vi "Asylum_Driver_LithographyObjects.vi"(4 "Abort Notifier":refnum<notifier>, 5 "Writing Setpoint":dbl=0.1 format="%#_13g", 6 "Interpolation":dbl format="%#_13g", 7 "Move Setpoint":dbl=-1.3 format="%#_13g", 8 "error in (no error)":errorcluster, 9 "Offsets":cluster{"X":dbl, "Y":dbl}, 10 "Lithography Data":T2(array[cluster]), 11 "Application":refnum<k7>) -> (0 "error out":errorcluster, 3 "Application Out":refnum<k7>)   [LabVIEW 2019]
uses:
  <userlib>/LevyLab/Relay Box/Typedefs/Resistor--enum.ctl
  <userlib>/LevyLab/Relay Box/Relay-Box.lvclass
panel:
  out "min value":dbl
  out "max value":dbl
  out "XY Graph":cluster{"X":dbl[], "Y":dbl[]}[](graph)
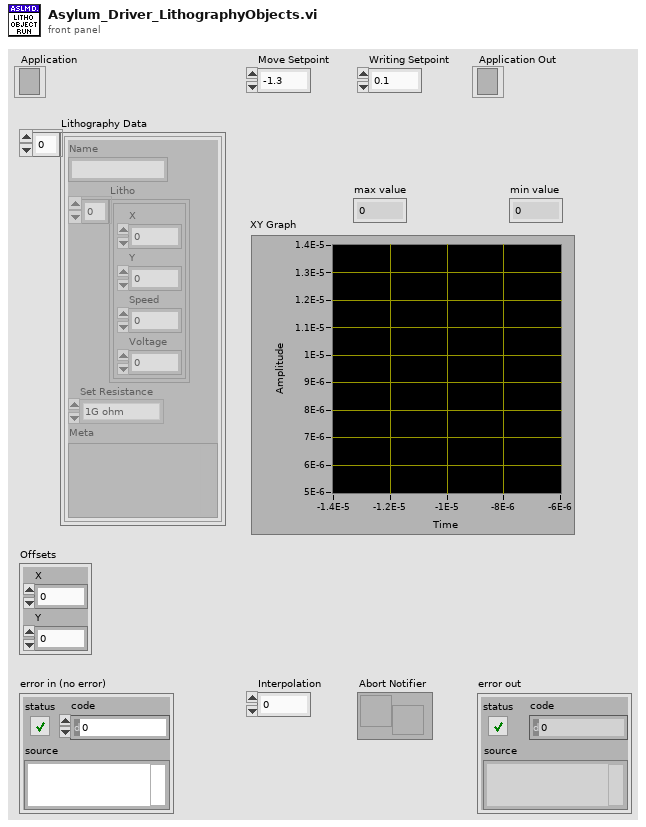
[diagram p1: front panel]
types:
  T1 = typedef "Relay-Box.lvclass/Resistor--enum.ctl" = enum16{"open", "discharge tip", "0 ohms", "100k ohm", "10M ohm", "1G ohm"}
  T2 = cluster{"Name":string, "Litho":cluster{"X":dbl, "Y":dbl, "Speed":dbl, "Voltage":dbl}[], "Set Resistance":T1, "Meta":variant}[]
  T3 = cluster{"X":dbl, "Y":dbl, "Speed":dbl, "Voltage":dbl}[]
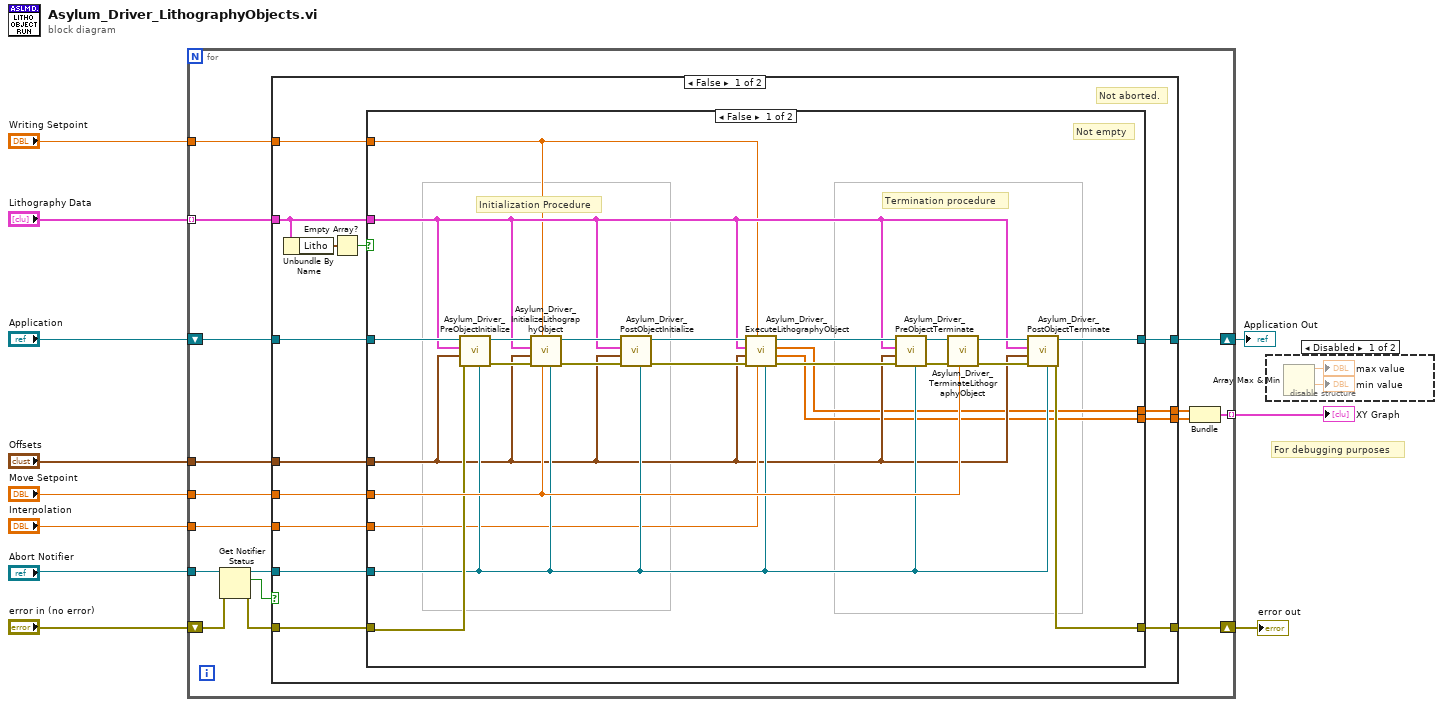
[diagram p0: block diagram]
diagram:
  # "For debugging purposes"
  n1 = for {
    tunnel: "Lithography Data" -> [w21] mode=indexing
    tunnel: "Offsets" -> [w23]
    shift-right: [w27] -> w10
    shift-left: "error in (no error)" -> [w26]
    tunnel: "Interpolation" -> [w24]
    tunnel: "Move Setpoint" -> [w20]
    tunnel: "Writing Setpoint" -> [w19]
    shift-right: [w18] -> w2
    shift-left: "Application" -> [w22]
    tunnel: "Abort Notifier" -> [w17]
    tunnel: [w12] -> w1 mode=indexing
    n2 = Get Notifier Status(notifier=w17, error in (no error)=w26) -> (notifier out=w15:refnum<notifier>, current notification=w16:bool, error out=w25:errorcluster)  [unwired: 2 out]
    n3 = case shown="False" w16 {
      tunnel: w25 -> [w41 w69]
      tunnel: [w40 w69] -> w27
      tunnel: w24 -> [w39 _]
      tunnel: w23 -> [w38 _]
      tunnel: w22 -> [w37 w68]
      tunnel: w21 -> [w35 _]
      tunnel: w20 -> [w33 _]
      tunnel: w19 -> [w32 _]
      tunnel: [w31 w68] -> w18
      tunnel: w15 -> [w30 _]
      tunnel: [w29 _] -> w14
      tunnel: [w28 _] -> w13
      frame False {
        # "Not aborted."
        n4 = Unbundle By Name(w35) -> ("Litho"=w34:T3)
        n5 = Empty Array?(array=w34) -> (empty?=w36:bool)
        n6 = case shown="False" w36 {
          tunnel: w41 -> [w54 w67]
          tunnel: w39 -> [w47 _]
          tunnel: [w53 w67] -> w40
          tunnel: w35 -> [w46 _]
          tunnel: w38 -> [w45 _]
          tunnel: w37 -> [w63 w66]
          tunnel: w33 -> [w65 _]
          tunnel: w32 -> [w44 _]
          tunnel: [w55 w66] -> w31
          tunnel: w30 -> [w48 _]
          tunnel: [w43 _] -> w29
          tunnel: [w42 _] -> w28
          frame False {
            # "Initialization Procedure"
            # "Termination procedure"
            # "Not empty"
            n7 = call "Asylum_Driver_PreObjectInitialize.vi"("Abort Notifier"=w48, "error in (no error)"=w54, "Offsets"=w45, "Pattern Data"=w46, "Application In"=w63) -> ("error out"=w64:errorcluster, "Application Out"=w60:refnum<k7>)  [unwired: 5 in]
            n8 = call "Asylum_Driver_InitializeLithographyObject.vi"("Abort Notifier"=w48, "Z Move Setpoint"=w65, "Z Write Setpoint"=w44, "error in (no error)"=w64, "Offsets"=w45, "Pattern Data"=w46, "Application"=w60) -> ("error out"=w62:errorcluster, "Application"=w61:refnum<k7>)  [unwired: 3 in]
            n9 = call "Asylum_Driver_PostObjectInitialize.vi"("Abort Notifier"=w48, "error in (no error)"=w62, "Offsets"=w45, "Pattern Data"=w46, "Application In"=w61) -> ("error out"=w49:errorcluster, "Application Out"=w52:refnum<k7>)  [unwired: 5 in]
            n10 = call "Asylum_Driver_ExecuteLithographyObject.vi"("Abort Notifier"=w48, "Interpolation"=w47, "Writing Setpoint"=w44, "error in (no error)"=w49, "Offsets"=w45, "Pattern Data"=w46, "Application In"=w52) -> ("error out"=w50:errorcluster, "Y"=w42:dbl[], "X"=w43:dbl[], "Application Out"=w51:refnum<k7>)  [unwired: 1 in]
            n11 = call "Asylum_Driver_PreObjectTerminate.vi"("Abort Notifier"=w48, "error in (no error)"=w50, "Offsets"=w45, "Pattern Data"=w46, "Application In"=w51) -> ("error out"=w58:errorcluster, "Application Out"=w59:refnum<k7>)  [unwired: 5 in]
            n12 = call "Asylum_Driver_TerminateLithographyObject.vi"("Z Move Setpoint"=w65, "error in (no error)"=w58, "Application"=w59) -> ("error out"=w56:errorcluster, "Application Out"=w57:refnum<k7>)  [unwired: 7 in]
            n13 = call "Asylum_Driver_PostObjectTerminate.vi"("Abort Notifier"=w48, "error in (no error)"=w56, "Offsets"=w45, "Pattern Data"=w46, "Application In"=w57) -> ("error out"=w53:errorcluster, "Application Out"=w55:refnum<k7>)  [unwired: 5 in]
          }
          frame True {
            # "Empty object. Dont do anything"
          }
        }
      }
      frame True {
        # "Previous Abort Sequence:\nWe would press Run, Done, on the AFM_Lithography VI and then press stop in the asylum software. \n\nNew Abort Sequence:\nRun (already called)\nDone = Abort (we call that through a notifier)\nStop = we call this when abort is signaled. (this is in the AFM software itself)\n\nThe rest of the lithography objects will be ignored."
        # "Aborted. Dont do anything for the rest of the sequence."
      }
    }
    n14 = Bundle("X"=w14, "Y"=w13) -> (w12:cluster{"X":dbl[], "Y":dbl[]})  [unwired: 1 in]
  }
  "error out" <- w10
  "Application Out" <- w2
  "XY Graph" <- w1
  n15 = disable-structure shown="Disabled" {
    frame Disabled {
      n16 = Array Max & Min() -> (max value=→"max value":dbl, min value=→"min value":dbl)  [unwired: 1 in, 2 out]
    }
    frame Enabled {
    }
  }
